vi "Pulse Width Math.vi"(11 "Pulse Width In":u32) -> (3 "Numeric":i32)   [LabVIEW 2014]
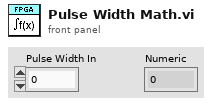
[diagram p1: front panel]
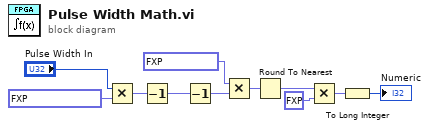
[diagram p0: block diagram]
diagram:
  n1 = Multiply(x="Pulse Width In", y=fxp<+,8,-5> 0.0169677734375) -> (x*y=w2:fxp<+,40,27>)
  n2 = Decrement(x=w2) -> (x-1=w1:fxp<+/-,41,28>)
  n3 = Decrement(x=w1) -> (x-1=w4:fxp<+/-,41,28>)
  n4 = Multiply(x=fxp<+,8,-2> 0.2001953125 ("frequency (periods/tick)"), y=w4) -> (x*y=w6:fxp<+/-,48,25>)
  n5 = Round To Nearest(number=w6) -> (nearest integer value=w7:fxp<+,24,24>)
  n6 = Multiply(x=w7, y=fxp<+,3,3> 5.0 ("frequency (periods/tick)")) -> (x*y=w8:fxp<+,27,27>)
  n7 = To Long Integer(number=w8) -> (32bit integer=→"Numeric":i32)
